vi "Wheel of Doom State.vi"() -> ()   [LabVIEW 2019]
uses:
  Wheel of Doom Slot State.ctl
panel:
  out "Current Slot":u32
  in  "Shoot 1":bool
  in  "Request Stop?":bool
  in  "Slot States":T1[](array[typedef])
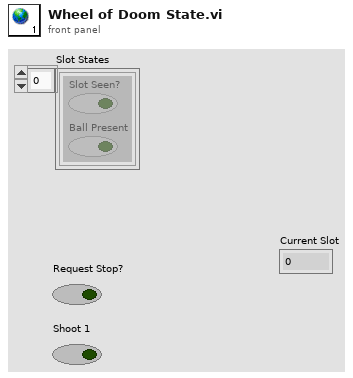
[diagram p1: front panel]
types:
  T1 = typedef "Wheel of Doom Slot State.ctl" = cluster{"Slot Seen?":bool, "Ball Present":bool}
diagram:
